vi "NI VeriStand - Close UDP Channel Streaming Session.vi"(8 "error in (no error)":errorcluster, 11 "UDPChannelStreamSession in":T1) -> (0 "error out":errorcluster)   [LabVIEW 2020, in "NI_VS Workspace ExecutionAPI.lvlib"]
doc: "Closes a UDP channel streaming session."
uses:
  <vilib>/NI VeriStand/Execution/Workspace/NI_VS Workspace ExecutionAPI.lvlib
  <vilib>/NI VeriStand/Execution/Workspace/UDPChannelStreamSession.ctl
  NationalInstruments.VeriStand.ClientAPI
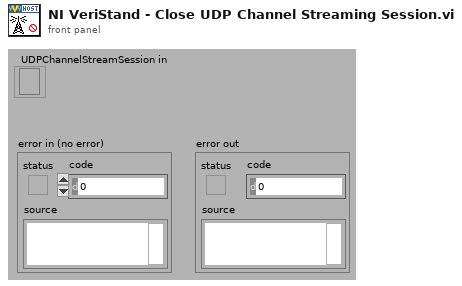
[diagram p1: front panel]
types:
  T1 = typedef "NI_VS Workspace ExecutionAPI.lvlib/UDPChannelStreamSession.ctl" = refnum<k24>
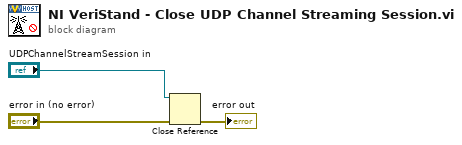
[diagram p0: block diagram]
diagram:
  n1 = Close Reference(reference="UDPChannelStreamSession in", error in (no error)="error in (no error)") -> (error out=→"error out":errorcluster)
